vi "Try Parse.vi"(0 "SA Path in":refnum<class "SA Abstract Path.lvclass">, 5 "Config Row":string[](array[string]), 11 "error in":errorcluster) -> (4 "SA Path out":refnum<class "SA Abstract Path.lvclass">, 6 "Is of type?":bool, 15 "error out":errorcluster)   [LabVIEW 2023, in "RFFixtureCharact.Public.lvlib" / "SA Abstract Path.lvclass"]
uses:
  SA Abstract Path.lvclass
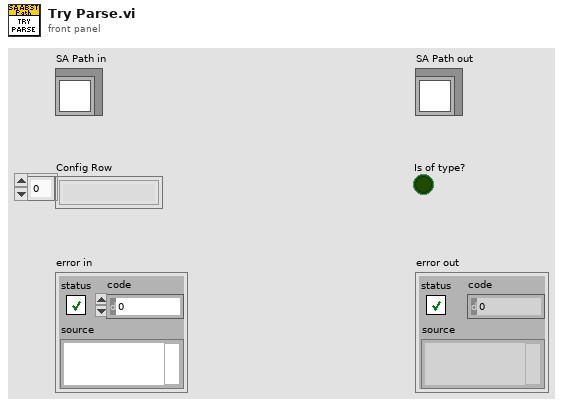
[diagram p1: front panel]
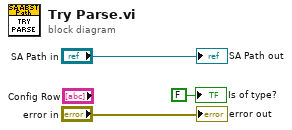
[diagram p0: block diagram]
diagram:
  "error out" <- "error in"
  "SA Path out" <- "SA Path in"
  "Is of type?" <- FALSE ("Is of type?")
